vi "Valve_SP.vi"(10 "Valve 1 SP":dbl=1.0) -> (2 "Output":u8[](array[numeric]))   [LabVIEW 2014]
panel:
  out "16bit integer":i16
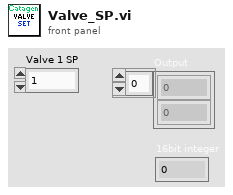
[diagram p1: front panel]
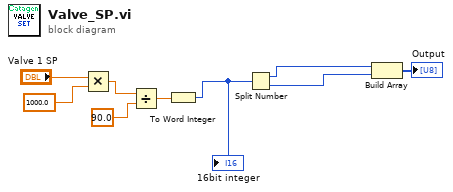
[diagram p0: block diagram]
diagram:
  n1 = Multiply(x="Valve 1 SP", y=1000.0) -> (x*y=w5:dbl)
  n2 = Divide(x=w5, y=90.0) -> (x/y=w2:dbl)
  n3 = To Word Integer(number=w2) -> (16bit integer=w1:i16)
  "16bit integer" <- w1
  n4 = Split Number(x=w1) -> (hi(x)=w9:u8, lo(x)=w8:u8)
  n5 = Build Array(w9, w8) -> (→"Output":u8[])
